vi "Version 1_Read Measurement Units.vi"(7 "Address (A)":string="A", 8 "error in":errorcluster, 10 "Software version (optional - wire for speed)":u8, 11 "VISA Session In":refnum<visa-resource-name>="Alicat") -> (0 "error out":errorcluster, 1 "Measurement Units - WILL NOT WORK WITH REV 6 AND ABOVE":T2, 3 "VISA Session Out":refnum<visa-resource-name>)   [LabVIEW 2016]
panel:
  out "Measurement Units Intermediate\n(older revisions)":T1={"Pressure Units"=0, "Mass Units"=0, "Temperature Units"=0, "Volume Units"=0, "Totalizer Units"=15, "Totalizer Avg Units"=15} {"Totalizer Units" items=["CC", "uL", "L", "CI", "CF", "CM", "GAL", "mL", "uP", "Lbs", "N/A", "N/A", "N/A", "SCC", "SuL", "SL", "SCI", "SCF", "NCM", "Grams", "Kg", "Lbs", "mg", "SCM", "SmL", "KSCF"]; "Totalizer Avg Units" items=["CCM", "uLPM", "LPM", "CIM", "CFM", "CM/M", "GAL/M", "mLPM", "uP/M", "Lbs/M", "N/A", "N/A", "N/A", "SCCM", "SuLPM", "SLPM", "SCIM", "SCFM", "NCM/M", "Grams/M", "Kg/M", "Lbs/M", "mg/M", "SCM/M", "SmLPM", "KSCFM"]; "Volume Units" items=["CCM"=0, "CCH"=64, "uLPM"=256, "LPS"=320, "LPM"=512, "CM/D"=576, "CIM"=768, "Percent"=832, "CFH"=1024, "Kg/M"=1088, "CM/H"=1280, "Kg/H"=1344, "CFM"=1536, "mLPS"=1600, "GPM"=1792, "CCS"=1856, "GPH"=2048, "mLPH"=2112, "Grams/S"=2304, "Lbs/H"=2368, "Grams/M"=2560, "Grams/H"=2816, "mg/M"=3072, "LPH"=3328, "oz/S"=3584, "mLPM"=3840]; "Temperature Units" items=["C"=0, "K"=16, "F"=32, "R"=48]; "Mass Units" items=["SCCM"=0, "SLPH"=128, "SuLPM"=4096, "SmLPM"=4224, "SLPM"=8192, "Grams/S"=8320, "SCIM"=12288, "SCM/H"=12416, "SCFH"=16384, "SCCH"=16512, "NCM/H"=20480, "NLPH"=20608, "SCFM"=24576, "NLPS"=24704, "Grams/M"=28672, "SCM/D"=28800, "Grams/H"=32768, "NmLPM"=32896, "Kg/M"=36864, "SCCS"=36992, "Kg/H"=40960, "NmLPH"=41088, "Lbs/M"=45056, "SLPS"=45184, "Lbs/H"=49152, "SmLPS"=49280, "mg/M"=53248, "mg/S"=53376, "NLPM"=57344, "NCCM"=61440]; "Pressure Units" items=["PSI", "PSI", "Torr", "Bar", "mBar", "Pascal", "KPa", "MPa", "inHg", "mmHg", "inH2O", "PSID", "mTorr", "cmH2O", "Kg/CM2", "mmH2O"]}
  # "Newer units of measure not included"
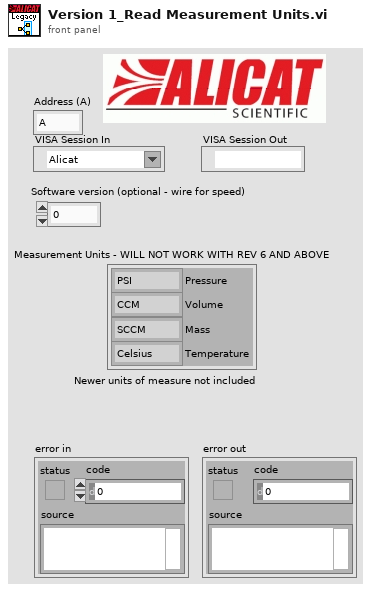
[diagram p1: front panel]
types:
  T1 = cluster{"Pressure Units":i32, "Mass Units":i32, "Temperature Units":i32, "Volume Units":i32, "Totalizer Units":u16, "Totalizer Avg Units":u16}
  T2 = cluster{"Pressure":enum8{"PSI", "PSI.", "Torr", "Bar", "mBar", "Pascal", "KPa", "MPa", "inHg", "mmHg", "inH2O", "PSID", "mTorr", "cmH2O", "Kg/CM2", "mmH2O"}, "Volume":enum8{"CCM", "CCH", "uLPM", "LPS", "LPM", "CM/D", "CIM", "Percent", "CFH", "Kg/M", "CM/H", "Kg/H", "CFM", "mLPS", "GPM", "CCS", "GPH", "mLPH", "Grams/S", "Lbs/H", "Grams/M", "Reserved (1)", "Grams/H", "Reserved (2)", "mg/M", "Reserved (3)"}, "Mass":enum32{"SCCM", "SLPH", "SuLPM", "SmLPM", "SLPM", "Grams/S", "SCIM", "SCM/H", "SCFH", "SCCH", "NCM/H", "NLPH", "SCFM", "NLPS", "Grams/M", "SCM/D", "Grams/H", "NmLPM", "Kg/M", "SCCS", "Kg/H", "NmLPH", "Lbs/M", "SLPS", "Lbs/H", "Reserved"}, "Temperature":enum8{"Celsius", "Kelvin", "Fahrenheit", "Rankin"}}
  T3 = enum8{"Celsius", "Kelvin", "Fahrenheit", "Rankin"}
  T4 = enum8{"PSI", "PSI.", "Torr", "Bar", "mBar", "Pascal", "KPa", "MPa", "inHg", "mmHg", "inH2O", "PSID", "mTorr", "cmH2O", "Kg/CM2", "mmH2O"}
  T5 = enum8{"CCM", "CCH", "uLPM", "LPS", "LPM", "CM/D", "CIM", "Percent", "CFH", "Kg/M", "CM/H", "Kg/H", "CFM", "mLPS", "GPM", "CCS", "GPH", "mLPH", "Grams/S", "Lbs/H", "Grams/M", "Reserved (1)", "Grams/H", "Reserved (2)", "mg/M", "Reserved (3)"}
  T6 = enum32{"SCCM", "SLPH", "SuLPM", "SmLPM", "SLPM", "Grams/S", "SCIM", "SCM/H", "SCFH", "SCCH", "NCM/H", "NLPH", "SCFM", "NLPS", "Grams/M", "SCM/D", "Grams/H", "NmLPM", "Kg/M", "SCCS", "Kg/H", "NmLPH", "Lbs/M", "SLPS", "Lbs/H", "Reserved"}
  T7 = cluster{"Pressure":i32, "Mass":i32, "Temperature":i32, "Volume":i32, "Totalizer Units":u16, "Totalizer Avg Units":u16}
  T8 = cluster{"Temperature":enum8{"Celsius", "Kelvin", "Fahrenheit", "Rankin"}}
  T9 = typedef "LVStringsAndValuesArrayTypeDef_I32.ctl" = cluster{"String":string, "Value":i32}[]
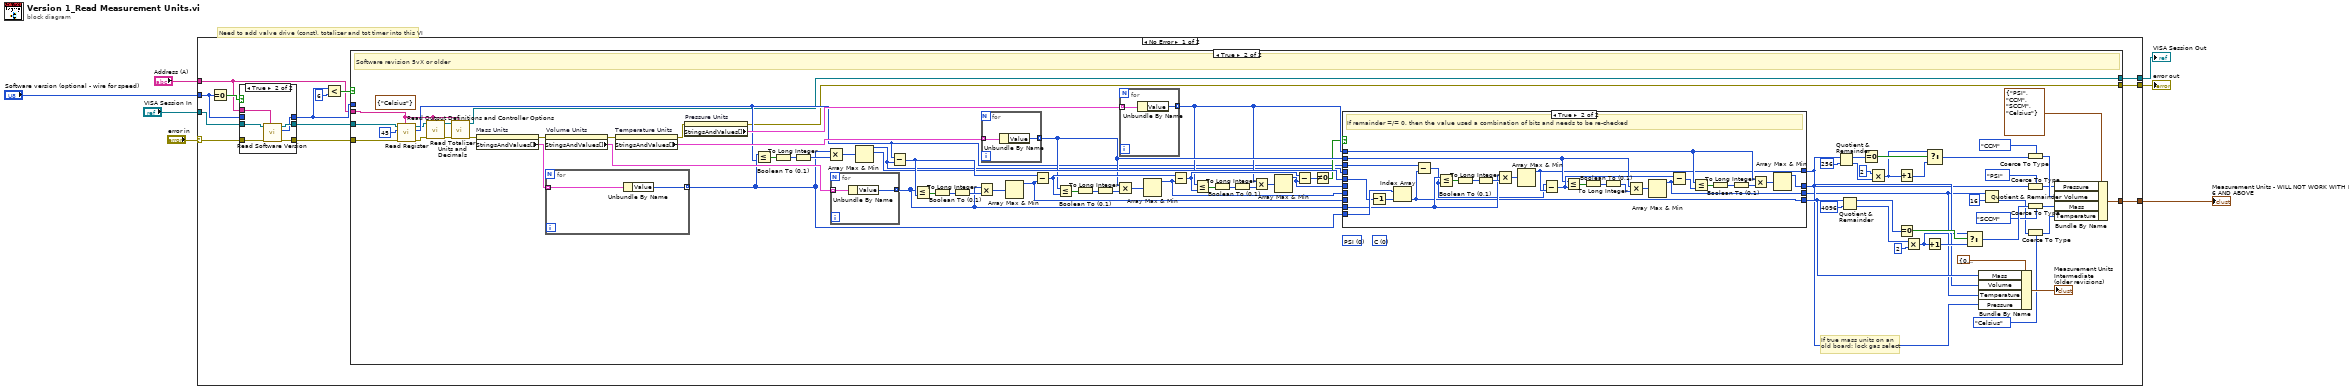
[diagram p0: block diagram]
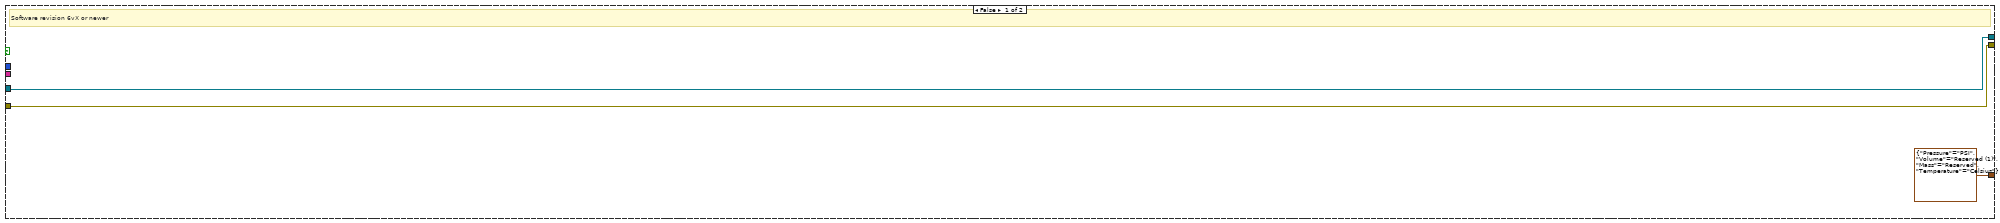
[diagram p3: hidden frame]
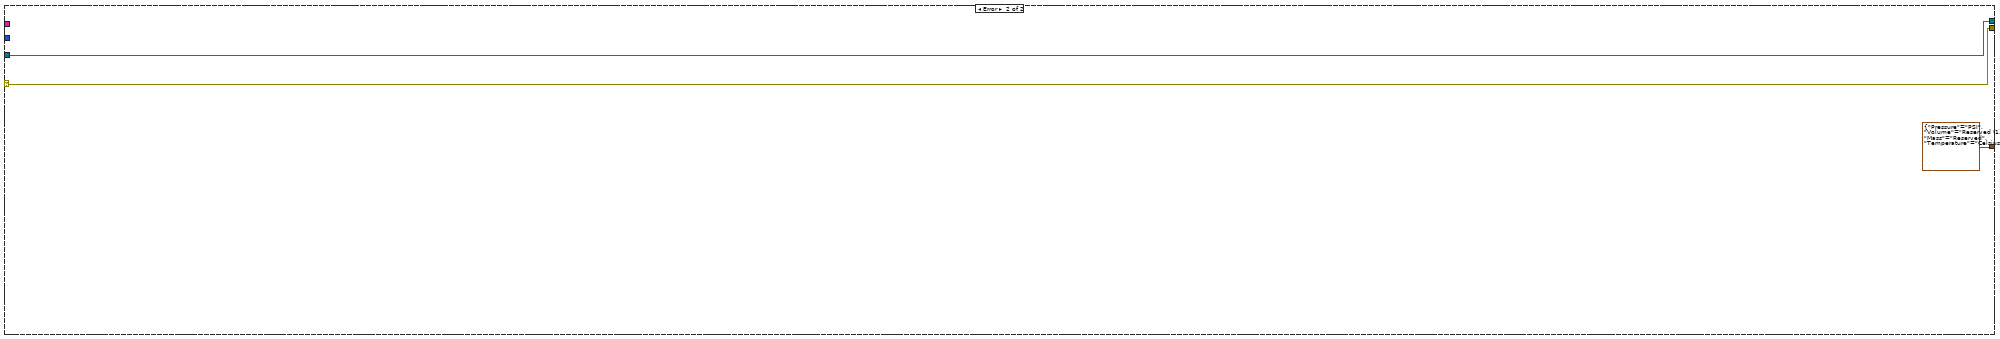
[diagram p5: hidden frame]
diagram:
  # "Need to add valve drive (const), totalizer and tot timer into this VI"
  n1 = case shown="No Error" "error in" {
    selector: "error in" -> [w11 w155]
    tunnel: [w20 w155] -> w2
    tunnel: "Software version (optional - wire for speed)" -> [w15 _]
    tunnel: "Address (A)" -> [w9 _]
    tunnel: "VISA Session In" -> [w10 w156]
    tunnel: [w18 w156] -> w3
    tunnel: [w8 T2 {"Pressure"=enum."PSI", "Volume"=enum."Reserved (1)", "Mass"=enum."Reserved", "Temperature"=enum."Celsius"} ("Measurement Units - WILL NOT WORK WITH REV 6 AND ABOVE")] -> w1
    frame No Error {
      n2 = Equal To 0?(x=w15) -> (x = 0?=w16:bool)
      n3 = case shown="True" w16 {
        tunnel: w11 -> [w22 w29]
        tunnel: w10 -> [w21 w28]
        tunnel: w9 -> [_ w27]
        tunnel: [w22 w26] -> w12
        tunnel: [w21 w25] -> w13
        tunnel: [w23 w24] -> w14
        tunnel: w15 -> [w23 _]
        frame False {
        }
        frame True {
          n4 = call "Read Software Version.vi"("Unit ID (A)"=w27, "error in"=w29, "VISA Session In"=w28) -> ("error out"=w26:errorcluster, "Software Version"=w24:u8, "VISA Session Out"=w25:refnum<visa-resource-name>)  [unwired: 6 in]
        }
      }
      n5 = Less?(x=w14, y=u8 6) -> (x < y?=w19:bool)
      n6 = case shown="True" w19 {
        tunnel: w12 -> [w31 w76]
        tunnel: [w31 w66] -> w20
        tunnel: w14 -> [_ _]
        tunnel: w13 -> [w30 w77]
        tunnel: w9 -> [_ w68]
        tunnel: [w30 w73] -> w18
        tunnel: [T2 {"Pressure"=enum."PSI", "Volume"=enum."Reserved (1)", "Mass"=enum."Reserved", "Temperature"=enum."Celsius"} ("Measurement Units - WILL NOT WORK WITH REV 6 AND ABOVE") w57] -> w8
        frame False {
          # "Software revision 6vX or newer"
        }
        frame True {
          (unwired) T8 {"Temperature"=enum."Celsius"} ("Measurement Units - WILL NOT WORK WITH REV 6 AND ABOVE")
          (unwired) 0 items=["PSI", "PSI", "Torr", "Bar", "mBar", "Pascal", "KPa", "MPa", "inHg", "mmHg", "inH2O", "PSID", "mTorr", "cmH2O", "Kg/CM2", "mmH2O"] ("Pressure")
          (unwired) 0 items=["C"=0, "K"=16, "F"=32, "R"=48] ("Temperature")
          # "If true mass units on an \nold board: lock gas select"
          # "Software revision 5vX or older"
          n7 = call "Read Register.vi"("Unit ID (A)"=w68, "error in"=w76, "Register address"=u16 45, "VISA Session In"=w77) -> ("error out"=w72:errorcluster, "Register Value (I32)"=w75:i32, "VISA Session Out"=w70:refnum<visa-resource-name>)  [unwired: 5 in]
          n8 = call "Read Output Definitions and Controller Options.vi"("Unit ID (A)"=w68, "error in"=w72, "VISA Session In"=w70) -> ("error out"=w71:errorcluster, "VISA Session Out"=w69:refnum<visa-resource-name>)  [unwired: 5 in, 2 out]
          n9 = call "Read Totalizer Units and Decimals.vi"("Unit ID (A)"=w68, "error in"=w71, "VISA Session In"=w69) -> ("error out"=w74:errorcluster, "VISA Session Out"=w73:refnum<visa-resource-name>)  [unwired: 4 in, 3 out]
          n10 = property on="Mass Units" class="Ring (strict)"(error in=w74) -> (error out=w81:errorcluster, "StringsAndValues[]"=w115:T9)  [unwired: 1 in, 1 out]
          n11 = property on="Volume Units" class="Ring (strict)"(error in=w81) -> (error out=w80:errorcluster, "StringsAndValues[]"=w106:T9)  [unwired: 1 in, 1 out]
          n12 = for {
            tunnel: w115 -> [w153] mode=indexing
            tunnel: [w152] -> w91 mode=indexing
            n13 = Unbundle By Name(w153) -> ("Value"=w152:i32)
          }
          n14 = property on="Temperature Units" class="Ring (strict)"(error in=w80) -> (error out=w79:errorcluster, "StringsAndValues[]"=w104:T9)  [unwired: 1 in, 1 out]
          n15 = property on="Pressure Units" class="Ring (strict)"(error in=w79) -> (error out=w66:errorcluster, "StringsAndValues[]"=w95:T9)  [unwired: 1 in, 1 out]
          n16 = Less Or Equal?(x=w91, y=w75) -> (x <= y?=w114:bool[])
          n17 = Boolean To (0,1)(Boolean=w114) -> (0, 1=w113:i16[])
          n18 = To Long Integer(number=w113) -> (32bit integer=w112:i32[])
          n19 = Multiply(x=w91, y=w112) -> (x*y=w111:i32[])
          n20 = for {
            tunnel: w106 -> [w151] mode=indexing
            tunnel: [w150] -> w89 mode=indexing
            n21 = Unbundle By Name(w151) -> ("Value"=w150:i32)
          }
          n22 = Array Max & Min(array=w111) -> (max value=w85:i32, max index (indices)=w90:i32)  [unwired: 2 out]
          n23 = Subtract(x=w75, y=w85) -> (x-y=w105:i32)
          n24 = Less Or Equal?(x=w89, y=w105) -> (x <= y?=w107:bool[])
          n25 = Boolean To (0,1)(Boolean=w107) -> (0, 1=w108:i16[])
          n26 = To Long Integer(number=w108) -> (32bit integer=w109:i32[])
          n27 = Multiply(x=w89, y=w109) -> (x*y=w110:i32[])
          n28 = for {
            tunnel: w104 -> [w149] mode=indexing
            tunnel: [w148] -> w88 mode=indexing
            n29 = Unbundle By Name(w149) -> ("Value"=w148:i32)
          }
          n30 = Array Max & Min(array=w110) -> (max value=w84:i32)  [unwired: 3 out]
          n31 = Subtract(x=w105, y=w84) -> (x-y=w94:i32)
          n32 = Less Or Equal?(x=w88, y=w94) -> (x <= y?=w103:bool[])
          n33 = Boolean To (0,1)(Boolean=w103) -> (0, 1=w102:i16[])
          n34 = To Long Integer(number=w102) -> (32bit integer=w101:i32[])
          n35 = Multiply(x=w88, y=w101) -> (x*y=w100:i32[])
          n36 = for {
            tunnel: w95 -> [w147] mode=indexing
            tunnel: [w146] -> w87 mode=indexing
            n37 = Unbundle By Name(w147) -> ("Value"=w146:i32)
          }
          n38 = Array Max & Min(array=w100) -> (max value=w83:i32)  [unwired: 3 out]
          n39 = Subtract(x=w94, y=w83) -> (x-y=w93:i32)
          n40 = Less Or Equal?(x=w87, y=w93) -> (x <= y?=w96:bool[])
          n41 = Boolean To (0,1)(Boolean=w96) -> (0, 1=w97:i16[])
          n42 = To Long Integer(number=w97) -> (32bit integer=w98:i32[])
          n43 = Multiply(x=w87, y=w98) -> (x*y=w99:i32[])
          n44 = Array Max & Min(array=w99) -> (max value=w82:i32)  [unwired: 3 out]
          n45 = Subtract(x=w93, y=w82) -> (x-y=w92:i32)
          n46 = Not Equal To 0?(x=w92) -> (x != 0?=w86:bool)
          n47 = case shown="True" w86 {
            tunnel: w91 -> [_ w145]
            tunnel: w90 -> [_ w143]
            tunnel: w89 -> [_ w138]
            tunnel: w88 -> [_ w132]
            tunnel: w87 -> [_ w126]
            tunnel: w85 -> [w119 _]
            tunnel: w84 -> [w118 _]
            tunnel: w83 -> [w117 _]
            tunnel: w82 -> [w116 _]
            tunnel: [w119 w121] -> w64
            tunnel: [w118 w125] -> w50
            tunnel: [w117 w124] -> w43
            tunnel: [w116 w123] -> w45
            tunnel: w75 -> [_ w120]
            frame False {
            }
            frame True {
              # "If remainder =/= 0, then the value used a combination of bits and needs to be re-checked"
              n48 = Decrement(x=w143) -> (x-1=w144:i32)
              n49 = Index Array(array=w145, index=w144) -> (element=w121:i32)
              n50 = Subtract(x=w120, y=w121) -> (x-y=w122:i32)
              n51 = Less Or Equal?(x=w138, y=w122) -> (x <= y?=w142:bool[])
              n52 = Boolean To (0,1)(Boolean=w142) -> (0, 1=w141:i16[])
              n53 = To Long Integer(number=w141) -> (32bit integer=w140:i32[])
              n54 = Multiply(x=w138, y=w140) -> (x*y=w139:i32[])
              n55 = Array Max & Min(array=w139) -> (max value=w125:i32)  [unwired: 3 out]
              n56 = Subtract(x=w122, y=w125) -> (x-y=w133:i32)
              n57 = Less Or Equal?(x=w132, y=w133) -> (x <= y?=w134:bool[])
              n58 = Boolean To (0,1)(Boolean=w134) -> (0, 1=w135:i16[])
              n59 = To Long Integer(number=w135) -> (32bit integer=w136:i32[])
              n60 = Multiply(x=w132, y=w136) -> (x*y=w137:i32[])
              n61 = Array Max & Min(array=w137) -> (max value=w124:i32)  [unwired: 3 out]
              n62 = Subtract(x=w133, y=w124) -> (x-y=w127:i32)
              n63 = Less Or Equal?(x=w126, y=w127) -> (x <= y?=w131:bool[])
              n64 = Boolean To (0,1)(Boolean=w131) -> (0, 1=w130:i16[])
              n65 = To Long Integer(number=w130) -> (32bit integer=w129:i32[])
              n66 = Multiply(x=w126, y=w129) -> (x*y=w128:i32[])
              n67 = Array Max & Min(array=w128) -> (max value=w123:i32)  [unwired: 3 out]
            }
          }
          n68 = Quotient & Remainder(x=w50, y=256) -> (x-y*floor(x/y)=w52:i32, floor(x/y)=w37:i32)
          n69 = Quotient & Remainder(x=w64, y=4096) -> (x-y*floor(x/y)=w62:i32, floor(x/y)=w35:i32)
          n70 = Equal To 0?(x=w52) -> (x = 0?=w53:bool)
          n71 = Multiply(x=2 ("floor(x/y)"), y=w37) -> (x*y=w36:i32)
          n72 = Increment(x=w36) -> (x+1=w54:i32)
          n73 = Equal To 0?(x=w62) -> (x = 0?=w61:bool)
          n74 = Multiply(x=w35, y=2 ("floor(x/y)")) -> (x*y=w33:i32)
          n75 = Increment(x=w33) -> (x+1=w60:i32)
          n76 = Select(t=w36, s=w53, f=w54) -> (s? t:f=w48:i32)
          n77 = Select(t=w33, s=w61, f=w60) -> (s? t:f=w59:i32)
          n78 = Bundle By Name(cluster=T7 {"Pressure"=0, "Mass"=0, "Temperature"=0, "Volume"=0, "Totalizer Units"=15, "Totalizer Avg Units"=15} ("Measurement Units Intermediate\n(older revisions)"), "Mass"=w64, "Volume"=w50, "Temperature"=w43, "Pressure"=w45) -> (→"Measurement Units Intermediate\n(older revisions)":T7)
          n79 = Quotient & Remainder(x=w43, y=16) -> (floor(x/y)=w40:i32)  [unwired: 1 out]
          n80 = Coerce To Type(0:w48, 1:T5."CCM" ("Volume")) -> (2:w47:T5)
          n81 = Coerce To Type(0:w45, 1:T4."PSI" ("Pressure")) -> (2:w44:T4)
          n82 = Coerce To Type(0:w59, 1:T6."SCCM" ("Mass")) -> (2:w55:T6)
          n83 = Coerce To Type(0:w40, 1:T3."Celsius" ("Temperature")) -> (2:w39:T3)
          n84 = Bundle By Name(cluster=T2 {"Pressure"=enum."PSI", "Volume"=enum."CCM", "Mass"=enum."SCCM", "Temperature"=enum."Celsius"} ("Measurement Units - WILL NOT WORK WITH REV 6 AND ABOVE"), "Pressure"=w44, "Volume"=w47, "Mass"=w55, "Temperature"=w39) -> (w57:T2)
        }
      }
    }
    frame Error {
    }
  }
  "error out" <- w2
  "VISA Session Out" <- w3
  "Measurement Units - WILL NOT WORK WITH REV 6 AND ABOVE" <- w1
